vi "Sort Targets.vi"(11 "Filtered Array":T1(array[cluster])) -> (3 "Sorted Array":T1(array[cluster]))   [LabVIEW 2012]
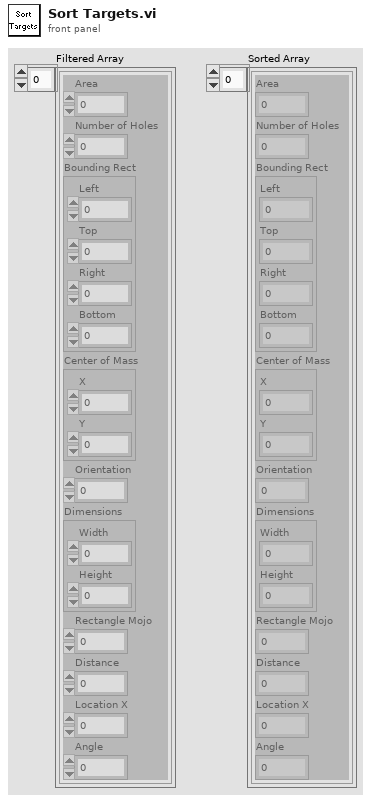
[diagram p1: front panel]
types:
  T1 = cluster{"Area":dbl, "Number of Holes":dbl, "Bounding Rect":cluster{"Left":dbl, "Top":dbl, "Right":dbl, "Bottom":dbl}, "Center of Mass":cluster{"X":dbl, "Y":dbl}, "Orientation":dbl, "Dimensions":cluster{"Width":dbl, "Height":dbl}, "Rectangle Mojo":dbl, "Distance":dbl, "Location X":dbl, "Angle":dbl}[]
  T2 = cluster{"Area":dbl, "Number of Holes":dbl, "Bounding Rect":cluster{"Left":dbl, "Top":dbl, "Right":dbl, "Bottom":dbl}, "Center of Mass":cluster{"X":dbl, "Y":dbl}, "Orientation":dbl, "Dimensions":cluster{"Width":dbl, "Height":dbl}, "Rectangle Mojo":dbl, "Distance":dbl, "Location X":dbl, "Angle":dbl}
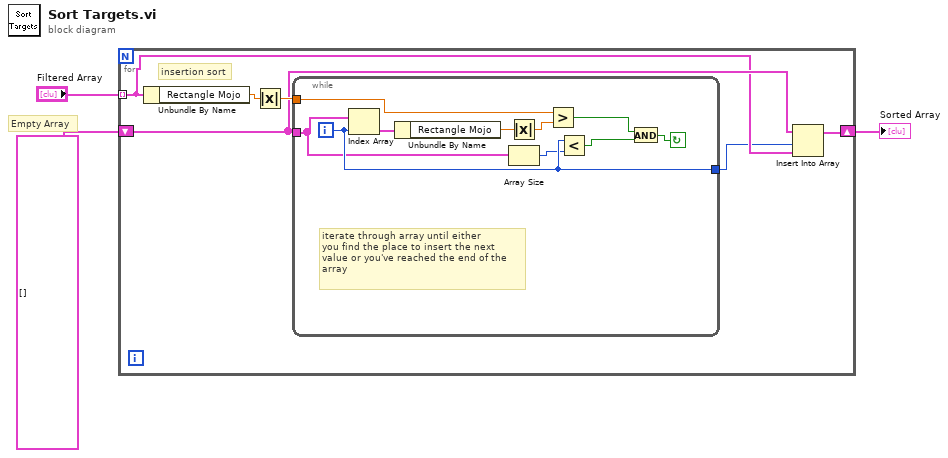
[diagram p0: block diagram]
diagram:
  # "Empty Array"
  n1 = for {
    tunnel: "Filtered Array" -> [w6] mode=indexing
    shift-right: [w5] -> w2
    shift-left: T1 [] ("Empty Array") -> [w7]
    # "insertion sort"
    n2 = Unbundle By Name(w6) -> ("Rectangle Mojo"=w9:dbl)
    n3 = Absolute Value(x=w9) -> (abs(x)=w8:dbl)
    n4 = while {
      tunnel: w7 -> [w14]
      tunnel: w8 -> [w17]
      tunnel: [w15] -> w4
      i -> [w15]
      stop <- w12 continue-if-true
      # "iterate through array until either\nyou find the place to insert the next\nvalue or you've reached the end of the\narray"
      n5 = Index Array(array=w14, index=w15) -> (element=w19:T2)
      n6 = Unbundle By Name(w19) -> ("Rectangle Mojo"=w18:dbl)
      n7 = Absolute Value(x=w18) -> (abs(x)=w16:dbl)
      n8 = Array Size(array=w14) -> (size(s)=w13:i32)
      n9 = Greater?(x=w17, y=w16) -> (0:w10:bool)
      n10 = Less?(x=w15, y=w13) -> (x < y?=w11:bool)
      n11 = And(x=w10, y=w11) -> (x .and. y?=w12:bool)
    }
    n12 = Insert Into Array(array=w7, index=w4, new element=w6) -> (w5:T1)
  }
  "Sorted Array" <- w2
